vi "Run Temperature Status.vi"(8 "error in (no error)":errorcluster, 11 "Channel in":refnum<class "Channel.lvclass">) -> (0 "error out":errorcluster, 3 "Channel out":refnum<class "Channel.lvclass">)   [LabVIEW 2018, in "Channel.lvclass"]
uses:
  Channel.lvclass
  State Machine/State Machine.lvclass/State Machine.ctl
  Channel.lvclass/Channel.ctl
  State Machine/State Machine.lvclass
  RxTx/RxTx.lvclass
  Interface/Interface.lvclass
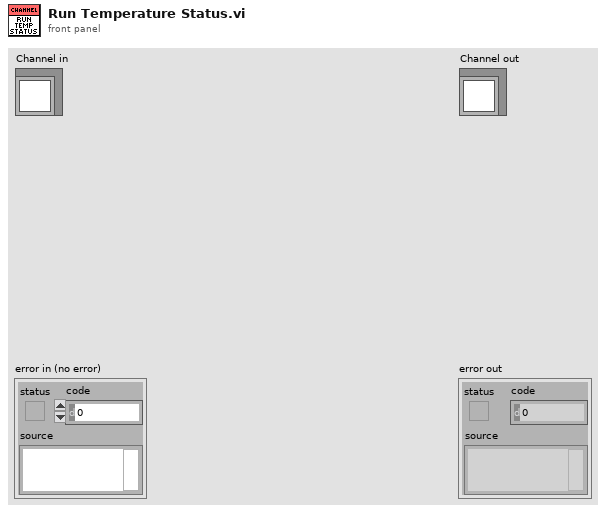
[diagram p1: front panel]
types:
  T1 = cluster{"CUBE_EXPOSURE_TIME":sgl, "CUBES_DONE":u16, "LAST_IMAGE_NAME":string, "DISK_SPACE":u16, "FRAMES_DONE":u16, "CCD_STATUS":string, "CURRENT_TEMPERATURE":i16, "TEMPERATURE_STATUS":string, "FRAME_EXPOSURE_TIME":u16, "CCD_ON_OFF":bool, "SERIAL_NUMBER":u16, "ACQUIRING":bool}
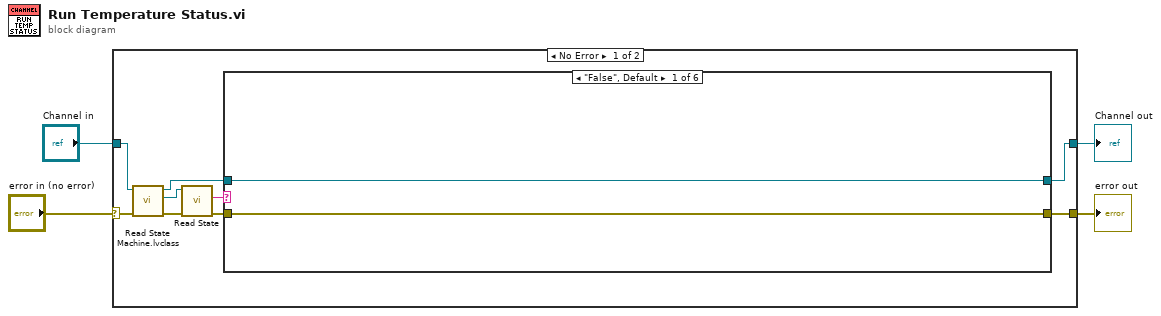
[diagram p0: block diagram]
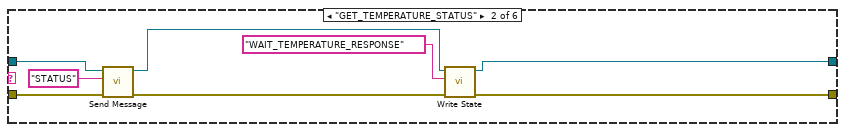
[diagram p2: hidden frame]
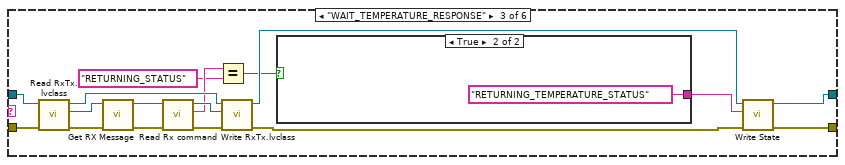
[diagram p3: hidden frame]
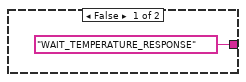
[diagram p4: hidden frame]
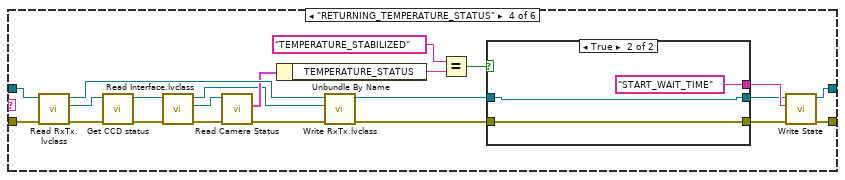
[diagram p5: hidden frame]
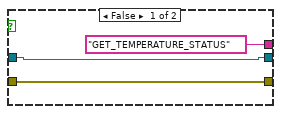
[diagram p6: hidden frame]
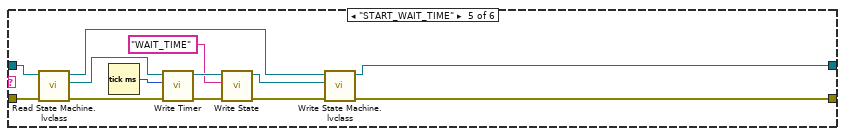
[diagram p7: hidden frame]
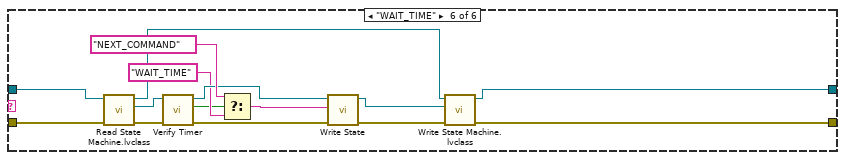
[diagram p8: hidden frame]
diagram:
  n1 = case shown="No Error" "error in (no error)" {
    selector: "error in (no error)" -> [w8 w100]
    tunnel: [w5 w100] -> w3
    tunnel: [w6 w99] -> w1
    tunnel: "Channel in" -> [w7 w99]
    frame No Error {
      n2 = call "Read State Machine.lvclass.vi"("error in (no error)"=w8, "Channel in"=w7) -> ("error out"=w12:errorcluster, "State Machine.lvclass"=w13:refnum<class "State Machine.lvclass">, "Channel out"=w10:refnum<class "Channel.lvclass">)  [unwired: 7 in]
      n3 = call-dynamic "Read State.vi"("error in (no error)"=w12, "State Machine in"=w13) -> ("error out"=w9:errorcluster, "State"=w11:string)  [unwired: 7 in, 1 out]
      n4 = case shown="\"False\", Default" w11 {
        tunnel: w10 -> [w15 w23 w27 w64 w83 w98]
        tunnel: w9 -> [w14 w22 w28 w63 w82 w97]
        tunnel: [w15 w18 w26 w60 w74 w94] -> w6
        tunnel: [w14 w17 w25 w61 w75 w95] -> w5
        frame "False", Default {
        }
        frame "GET_TEMPERATURE_STATUS" {
          n5 = call "Send Message.vi"("error in (no error)"=w22, "message"="STATUS", "Channel in"=w23) -> ("error out"=w19:errorcluster, "Channel out"=w20:refnum<class "Channel.lvclass">)  [unwired: 7 in]
          n6 = call "Write State.vi"("error in (no error)"=w19, "State"="WAIT_TEMPERATURE_RESPONSE" ("message"), "Channel in"=w20) -> ("error out"=w17:errorcluster, "Channel out"=w18:refnum<class "Channel.lvclass">)  [unwired: 7 in]
        }
        frame "WAIT_TEMPERATURE_RESPONSE" {
          n7 = call "Read RxTx.lvclass.vi"("error in (no error)"=w28, "Channel in"=w27) -> ("error out"=w38:errorcluster, "RxTx.lvclass"=w37:refnum<class "RxTx.lvclass">, "Channel out"=w34:refnum<class "Channel.lvclass">)  [unwired: 7 in]
          n8 = call "Get RX Message.vi"("error in (no error)"=w38, "RxTx in"=w37) -> ("error out"=w39:errorcluster, "RxTx out"=w40:refnum<class "RxTx.lvclass">)  [unwired: 8 in]
          n9 = call "Read Rx command.vi"("error in (no error)"=w39, "RxTx in"=w40) -> ("error out"=w36:errorcluster, "Rx Command"=w29:string, "RxTx out"=w35:refnum<class "RxTx.lvclass">)  [unwired: 7 in]
          n10 = Equal?(x=w29, y="RETURNING_STATUS") -> (x = y?=w31:bool)
          n11 = call "Write RxTx.lvclass.vi"("error in (no error)"=w36, "RxTx.lvclass"=w35, "Channel in"=w34) -> ("error out"=w32:errorcluster, "Channel out"=w33:refnum<class "Channel.lvclass">)  [unwired: 7 in]
          n12 = case shown="True" w31 {
            tunnel: ["WAIT_TEMPERATURE_RESPONSE" "RETURNING_TEMPERATURE_STATUS"] -> w30
            frame False {
            }
            frame True {
            }
          }
          n13 = call "Write State.vi"("error in (no error)"=w32, "State"=w30, "Channel in"=w33) -> ("error out"=w25:errorcluster, "Channel out"=w26:refnum<class "Channel.lvclass">)  [unwired: 7 in]
        }
        frame "RETURNING_TEMPERATURE_STATUS" {
          n14 = call "Read RxTx.lvclass.vi"("error in (no error)"=w63, "Channel in"=w64) -> ("error out"=w58:errorcluster, "RxTx.lvclass"=w59:refnum<class "RxTx.lvclass">, "Channel out"=w62:refnum<class "Channel.lvclass">)  [unwired: 7 in]
          n15 = call "Get CCD status.vi"("error in (no error)"=w58, "RxTx in"=w59) -> ("error out"=w56:errorcluster, "RxTx out"=w57:refnum<class "RxTx.lvclass">)  [unwired: 8 in]
          n16 = call "Read Interface.lvclass.vi"("error in (no error)"=w56, "RxTx in"=w57) -> ("error out"=w54:errorcluster, "Interface.lvclass"=w55:refnum<class "Interface.lvclass">, "RxTx out"=w47:refnum<class "RxTx.lvclass">)  [unwired: 7 in]
          n17 = call "Read Camera Status.vi"("error in (no error)"=w54, "Interface in"=w55) -> ("error out"=w48:errorcluster, "Camera Status"=w53:T1)  [unwired: 7 in, 1 out]
          n18 = Unbundle By Name(w53) -> ("TEMPERATURE_STATUS"=w52:string)
          n19 = call "Write RxTx.lvclass.vi"("error in (no error)"=w48, "RxTx.lvclass"=w47, "Channel in"=w62) -> ("error out"=w46:errorcluster, "Channel out"=w44:refnum<class "Channel.lvclass">)  [unwired: 7 in]
          n20 = Equal?(x="TEMPERATURE_STABILIZED" ("State"), y=w52) -> (x = y?=w50:bool)
          n21 = case shown="True" w50 {
            tunnel: ["GET_TEMPERATURE_STATUS" ("State") "START_WAIT_TIME" ("State")] -> w49
            tunnel: w46 -> [w66 w68]
            tunnel: [w66 w68] -> w45
            tunnel: w44 -> [w65 w69]
            tunnel: [w65 w69] -> w43
            frame False {
            }
            frame True {
            }
          }
          n22 = call "Write State.vi"("error in (no error)"=w45, "State"=w49, "Channel in"=w43) -> ("error out"=w61:errorcluster, "Channel out"=w60:refnum<class "Channel.lvclass">)  [unwired: 7 in]
        }
        frame "START_WAIT_TIME" {
          n23 = call "Read State Machine.lvclass.vi"("error in (no error)"=w82, "Channel in"=w83) -> ("error out"=w80:errorcluster, "State Machine.lvclass"=w81:refnum<class "State Machine.lvclass">, "Channel out"=w76:refnum<class "Channel.lvclass">)  [unwired: 7 in]
          n24 = Tick Count (ms)() -> (millisecond timer value=w77:u32)
          n25 = call "Write Timer.vi"("error in (no error)"=w80, "Timer"=w77, "State Machine in"=w81) -> ("error out"=w78:errorcluster, "State Machine out"=w79:refnum<class "State Machine.lvclass">)  [unwired: 7 in]
          n26 = call-dynamic "Write State.vi"("error in (no error)"=w78, "State"="WAIT_TIME", "State Machine in"=w79) -> ("error out"=w72:errorcluster, "State Machine out"=w73:refnum<class "State Machine.lvclass">)  [unwired: 7 in]
          n27 = call "Write State Machine.lvclass.vi"("error in (no error)"=w72, "State Machine.lvclass"=w73, "Channel in"=w76) -> ("error out"=w75:errorcluster, "Channel out"=w74:refnum<class "Channel.lvclass">)  [unwired: 7 in]
        }
        frame "WAIT_TIME" {
          n28 = call "Read State Machine.lvclass.vi"("error in (no error)"=w97, "Channel in"=w98) -> ("error out"=w90:errorcluster, "State Machine.lvclass"=w91:refnum<class "State Machine.lvclass">, "Channel out"=w96:refnum<class "Channel.lvclass">)  [unwired: 7 in]
          n29 = call "Verify Timer.vi"("error in (no error)"=w90, "State Machine in"=w91) -> ("error out"=w86:errorcluster, "Time out"=w84:bool, "State Machine out"=w87:refnum<class "State Machine.lvclass">)  [unwired: 6 in, 1 out]
          n30 = Select(t="NEXT_COMMAND", s=w84, f="WAIT_TIME") -> (s? t:f=w88:string)
          n31 = call-dynamic "Write State.vi"("error in (no error)"=w86, "State"=w88, "State Machine in"=w87) -> ("error out"=w92:errorcluster, "State Machine out"=w93:refnum<class "State Machine.lvclass">)  [unwired: 7 in]
          n32 = call "Write State Machine.lvclass.vi"("error in (no error)"=w92, "State Machine.lvclass"=w93, "Channel in"=w96) -> ("error out"=w95:errorcluster, "Channel out"=w94:refnum<class "Channel.lvclass">)  [unwired: 7 in]
        }
      }
    }
    frame Error {
    }
  }
  "error out" <- w3
  "Channel out" <- w1
